vi "Regression Solver.vi"() -> ()   [LabVIEW 2014]
doc: "Demonstrates how to use the linear, polynomial, exponential, and power Fitting VIs for selected data sets."
uses:
  <vilib>/Utility/error.llb/DialogType.ctl
  <vilib>/Analysis/NI_AALPro.lvlib
  <vilib>/gmath/NI_Gmath.lvlib
panel:
  in  "Fitting method":u16(ring) items=["Least Square", "Least Absolute Residual", "Bisquare"]
  out "Equation of fit":string
  out "XY Graph":T1(graph)
  in  "Display Precision":i32=3 min=0
  in  "Stop":bool
  out "Fitted Data":dbl[](array[numeric]) format="%#.6g"
  out "MSE":dbl format="%#.3g"
  in  "Data":dbl[][](array[numeric])=[[0.01, 0.0], [1.0, 2.700000047683716], [2.0, 7.400000095367432], [3.0, 30.0], [4.0, 80.0], [5.0, 220.0]] format="%#.6g"
  out "error information":string
  in  "Order":i32=2
  in  "Models":T2(radio)
  # "Overview: Demonstrates fitting data to linear, polynomial, exponential and power models with the Fitting VIs.\nRequirements: LabVIEW Full Development System\nInstructions: \n1. Run the VI. \n2. Select different Models and notice the changes to the graph and MSE.\n3. Click Stop to stop the VI."
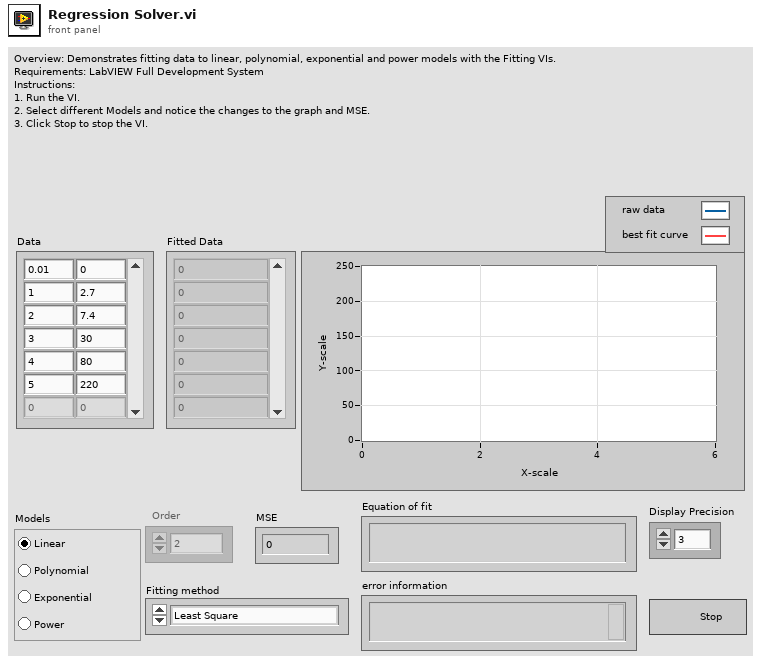
[diagram p1: front panel]
types:
  T1 = cluster{"Data":dbl[], "Best Exponential Fit":dbl[]}[]
  T2 = enum32{"Linear", "Polynomial", "Exponential", "Power"}
  T3 = enum8{"Enabled", "Disabled", "Disabled and Grayed Out"}
  T4 = enum16{"Linear", "Polynomial", "Exponential", "Power"}
  T5 = cluster{"amp min":dbl, "amp max":dbl, "damping min":dbl, "damping max":dbl, "offset min":dbl, "offset max":dbl}
  T6 = typedef "DialogType.ctl" = u16
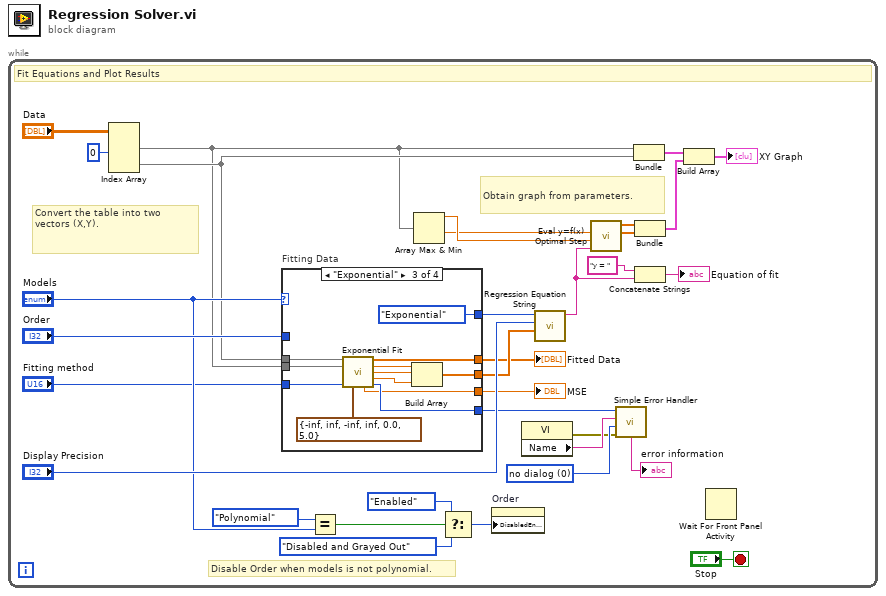
[diagram p0: block diagram]
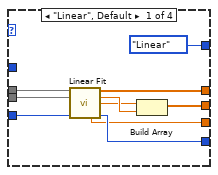
[diagram p2: hidden frame]
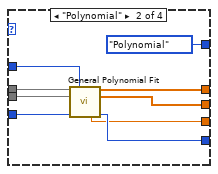
[diagram p3: hidden frame]
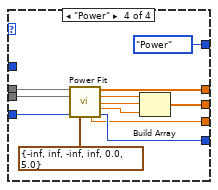
[diagram p4: hidden frame]
diagram:
  n1 = while {
    stop <- "Stop" stop-if-true
    w25 = T6 0 items=["no dialog", "OK message", "continue or stop message", "OK message + warnings", "continue/stop + warnings"] ("type of dialog (OK msg:1)")
    # "Convert the table into two vectors (X,Y)."
    # "Disable Order when models is not polynomial."
    # "Obtain graph from parameters."
    # "Fit Equations and Plot Results"
    n2 = Index Array(array="Data", index (col) #1=0 ("disabled index (col)")) -> (element #1=w10:dbl[], element #2=w11:dbl[])  [unwired: 3 in]
    n3 = case "Fitting Data" shown="\"Exponential\"" "Models" {
      tunnel: [w43 w52 w62 w75] -> w29
      tunnel: w11 -> [w42 w51 w63 w67]
      tunnel: w10 -> [w40 w50 w64 w76]
      tunnel: [w36 w49 w61 w74] -> w28
      tunnel: [w41 w48 w60 w73] -> w23
      tunnel: [w37 w47 w57 w70] -> w24
      tunnel: "Order" -> [_ w46 _ _]
      tunnel: "Fitting method" -> [w35 w45 w54 w68]
      tunnel: [T4."Linear" ("fit type") T4."Polynomial" ("fit type") T4."Exponential" ("fit type") T4."Power" ("fit type")] -> w4
      frame "Linear", Default {
        n4 = call <vilib>:"Linear Fit.vi"("Y"=w42, "X"=w40, "method"=w35) -> ("Best Linear Fit"=w41:dbl[], "slope"=w39:dbl, "intercept"=w38:dbl, "residue"=w36:dbl, "error"=w43:i32)  [unwired: 8 in]
        n5 = Build Array(w38, w39) -> (w37:dbl[])
      }
      frame "Polynomial" {
        n6 = call <vilib>:"General Polynomial Fit.vi"("Y"=w51, "polynomial order"=w46, "X"=w50, "method"=w45) -> ("Best Polynomial Fit"=w48:dbl[], "Polynomial Coefficients"=w47:dbl[], "residue"=w49:dbl, "error"=w52:i32)  [unwired: 8 in]
      }
      frame "Exponential" {
        n7 = call <vilib>:"Exponential Fit.vi"("Y"=w63, "X"=w64, "method"=w54, "parameter bounds"=T5 {"amp min"=-inf, "amp max"=inf, "damping min"=-inf, "damping max"=inf, "offset min"=0.0, "offset max"=5.0}) -> ("Best Exponential Fit"=w60:dbl[], "amplitude"=w58:dbl, "damping"=w59:dbl, "offset"=w56:dbl, "residue"=w61:dbl, "error"=w62:i32)  [unwired: 6 in]
        n8 = Build Array(w58, w59, w56) -> (w57:dbl[])
      }
      frame "Power" {
        n9 = call <vilib>:"Power Fit.vi"("Y"=w67, "X"=w76, "method"=w68, "parameter bounds"=T5 {"amp min"=-inf, "amp max"=inf, "damping min"=-inf, "damping max"=inf, "offset min"=0.0, "offset max"=5.0}) -> ("Best Power Fit"=w73:dbl[], "amplitude"=w71:dbl, "power"=w72:dbl, "offset"=w69:dbl, "residue"=w74:dbl, "error"=w75:i32)  [unwired: 6 in]
        n10 = Build Array(w71, w72, w69) -> (w70:dbl[])
      }
    }
    "Fitted Data" <- w23
    "MSE" <- w28
    n11 = Equal?(x=T2."Polynomial", y="Models") -> (x = y?=w20:bool)
    n12 = Array Max & Min(array=w10) -> (max value=w12:dbl, min value=w5:dbl)  [unwired: 2 out]
    n13 = Select(t=T3."Enabled" ("Disabled"), s=w20, f=T3."Disabled and Grayed Out" ("Disabled")) -> (s? t:f=w17:T3)
    n14 = property on="Order" class="DigNum (strict)"("DisabledEnum"=w17) -> ()  [unwired: 2 in, 2 out]
    n15 = property class="VI"() -> (error out=w1:errorcluster, "Name"=w2:string)  [unwired: 2 in, 1 out]
    n16 = call "Regression Equation String.vi"("coefficients"=w24, "precision"="Display Precision", "fit type"=w4) -> ("Formula"=w6:string)  [unwired: 8 in]
    n17 = call <vilib>:"Eval y=f(x) Optimal Step.vi"("formula"=w6, "end"=w12, "start"=w5) -> ("Y Values"=w15:dbl[], "X Values"=w16:dbl[])  [unwired: 2 in, 2 out]
    n18 = call <vilib>:"Simple Error Handler.vi"("error code (no error:0)"=w29, "error source (\" \")"=w2, "type of dialog (OK msg:1)"=w25, "error in (no error)"=w1) -> ("message"=→"error information":string)  [unwired: 1 in, 4 out]
    n19 = Bundle("Data"=w10, "Data"=w11) -> (w26:cluster{"Data":dbl[], "Data":dbl[]})  [unwired: 1 in]
    n20 = Bundle("X Values"=w16, "Y Values"=w15) -> (w22:cluster{"X Values":dbl[], "Y Values":dbl[]})  [unwired: 1 in]
    n21 = Concatenate Strings("y = " ("string"), w6) -> (→"Equation of fit":string)
    n22 = Build Array(w26, w22) -> (→"XY Graph":cluster{"X Values":dbl[], "Y Values":dbl[]}[])
    n23 = Wait For Front Panel Activity() -> ()  [unwired: 3 in, 1 out]
  }
